vi "LoadCommCfg.vi"(8 "error in (no error)":errorcluster, 10 "section (server name)":string, 11 "Server in":refnum<class "Server.lvclass">) -> (0 "error out":errorcluster, 3 "Server out":refnum<class "Server.lvclass">)   [LabVIEW 2018, in "Server.lvclass"]
uses:
  Server.lvclass
  Server.lvclass/Server.ctl
  <vilib>/Utility/config.llb/Read Key (I32).vi
  <vilib>/Utility/config.llb/Read Key (String).vi
  Comm/Stream/Stream.lvclass
  <vilib>/Utility/config.llb/NI_LVConfig.lvlib
panel:
  out "error commfile2":errorcluster
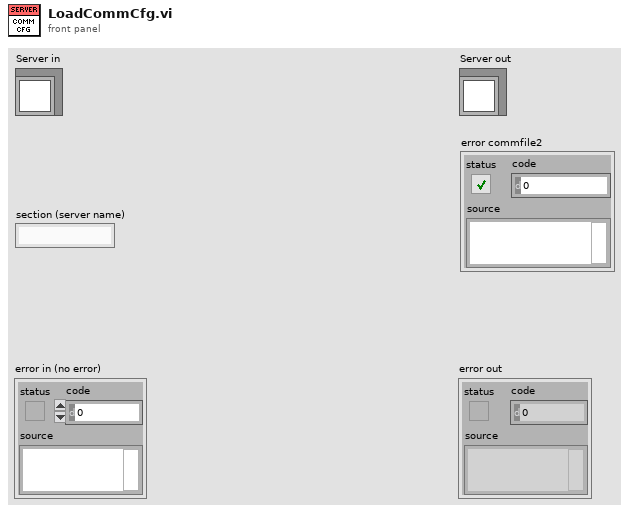
[diagram p1: front panel]
types:
  T1 = typedef "NI_LVConfig.lvlib/Config Data RefNum.ctl" = refnum<k1>
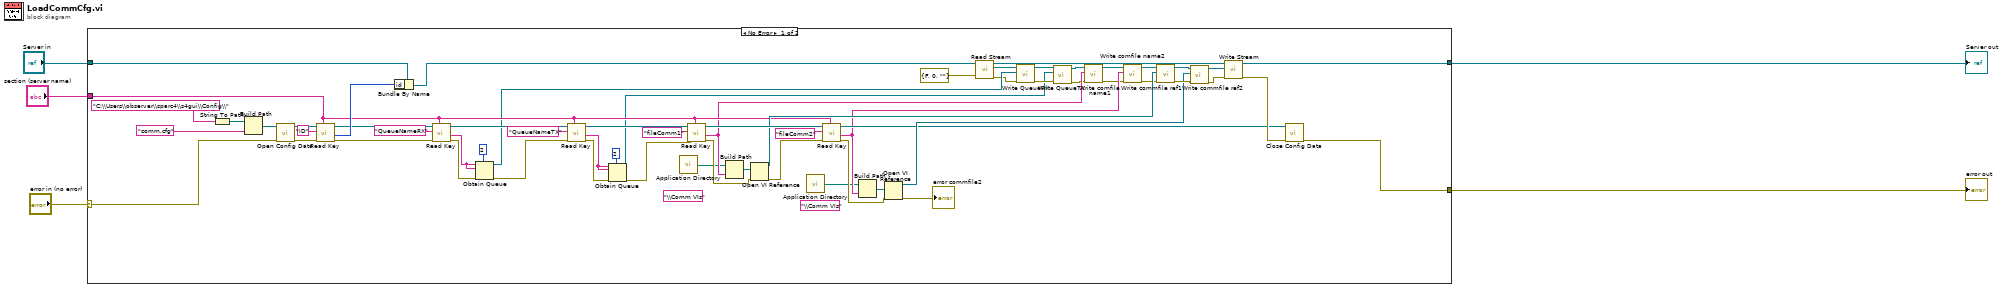
[diagram p0: block diagram]
diagram:
  n1 = case shown="No Error" "error in (no error)" {
    selector: "error in (no error)" -> [w63 w70]
    tunnel: [w60 w70] -> w4
    tunnel: [w48 w69] -> w2
    tunnel: "Server in" -> [w62 w69]
    tunnel: "section (server name)" -> [w31 _]
    frame No Error {
      (unwired) "\\Comm VIs" ("string")
      (unwired) "\\Comm VIs" ("string")
      n2 = String To Path(string="C:\\Users\\observer\\sparc4\\s4gui\\Config\\") -> (path=w6:path)
      n3 = Build Path(base path=w6, name or relative path="comm.cfg") -> (appended path=w68:path)
      n4 = call <vilib>:"Open Config Data.vi"("error in (no error)"=w63, "configuration file path"=w68) -> ("error out"=w65:errorcluster, "refnum"=w67:T1)  [unwired: 7 in, 1 out]
      n5 = call-poly <vilib>:"Read Key.vi"("section"=w31, "error in (no error)"=w65, "key"="ID", "refnum"=w67) -> ("error out"=w51:errorcluster, "value"=w61:i32, "refnum out"=w52:T1)  [unwired: 4 in, 1 out]
      n6 = Bundle By Name(cluster=w62, "id"=w61) -> (w50:refnum<class "Server.lvclass">)
      n7 = call-poly <vilib>:"Read Key.vi"("section"=w31, "error in (no error)"=w51, "key"="QueueNameRX", "refnum"=w52) -> ("error out"=w46:errorcluster, "value"=w58:string, "refnum out"=w57:T1)  [unwired: 4 in, 1 out]
      n8 = Obtain Queue(max queue size (-1, unlimited)=2, name (unnamed)=w58, element data type=w58, error in (no error)=w46) -> (queue out=w18:refnum<queue>, error out=w45:errorcluster)  [unwired: 1 in, 1 out]
      n9 = call-poly <vilib>:"Read Key.vi"("section"=w31, "error in (no error)"=w45, "key"="QueueNameTX", "refnum"=w57) -> ("error out"=w44:errorcluster, "value"=w59:string, "refnum out"=w20:T1)  [unwired: 4 in, 1 out]
      n10 = Obtain Queue(max queue size (-1, unlimited)=2, name (unnamed)=w59, element data type=w59, error in (no error)=w44) -> (queue out=w12:refnum<queue>, error out=w35:errorcluster)  [unwired: 1 in, 1 out]
      n11 = call <vilib>:"Application Directory.vi"() -> ("Application Directory"=w9:path)
      n12 = call-poly <vilib>:"Read Key.vi"("section"=w31, "error in (no error)"=w35, "key"="fileComm1", "refnum"=w20) -> ("error out"=w34:errorcluster, "value"=w26:string, "refnum out"=w43:T1)  [unwired: 4 in, 1 out]
      n13 = Build Path(base path=w9, name or relative path=w26) -> (appended path=w36:path)
      n14 = Open VI Reference(vi path=w36, error in (no error)=w34) -> (vi reference=w32:refnum<vi>, error out=w33:errorcluster)  [unwired: 4 in]
      n15 = call <vilib>:"Application Directory.vi"() -> ("Application Directory"=w8:path)
      n16 = call-poly <vilib>:"Read Key.vi"("section"=w31, "error in (no error)"=w33, "key"="fileComm2", "refnum"=w43) -> ("error out"=w29:errorcluster, "value"=w25:string, "refnum out"=w27:T1)  [unwired: 4 in, 1 out]
      n17 = Build Path(base path=w8, name or relative path=w25) -> (appended path=w30:path)
      n18 = Open VI Reference(vi path=w30, error in (no error)=w29) -> (vi reference=w28:refnum<vi>, error out=→"error commfile2":errorcluster)  [unwired: 4 in]
      n19 = call-dynamic "Read Stream.vi"("error in (no error)"=errorcluster {"status"=FALSE, "code"=0, "source"=""}, "Server in"=w50) -> ("error out"=w17:errorcluster, "Stream.lvclass"=w19:refnum<class "Stream.lvclass">, "Server out"=w49:refnum<class "Server.lvclass">)  [unwired: 7 in]
      n20 = call-dynamic "Write QueueRX.vi"("error in (no error)"=w17, "queue RX"=w18, "Stream in"=w19) -> ("error out"=w15:errorcluster, "Stream out"=w16:refnum<class "Stream.lvclass">)  [unwired: 7 in]
      n21 = call-dynamic "Write QueueTX.vi"("error in (no error)"=w15, "queue TX"=w12, "Stream in"=w16) -> ("error out"=w13:errorcluster, "Stream out"=w14:refnum<class "Stream.lvclass">)  [unwired: 7 in]
      n22 = call-dynamic "Write comfile name1.vi"("error in (no error)"=w13, "comfile name1"=w26, "Stream in"=w14) -> ("error out"=w22:errorcluster, "Stream out"=w24:refnum<class "Stream.lvclass">)  [unwired: 7 in]
      n23 = call-dynamic "Write comfile name2.vi"("error in (no error)"=w22, "comfile name2"=w25, "Stream in"=w24) -> ("error out"=w21:errorcluster, "Stream out"=w23:refnum<class "Stream.lvclass">)  [unwired: 7 in]
      n24 = call-dynamic "Write commfile ref1.vi"("error in (no error)"=w21, "commfile ref1"=w32, "Stream in"=w23) -> ("error out"=w38:errorcluster, "Stream out"=w40:refnum<class "Stream.lvclass">)  [unwired: 7 in]
      n25 = call-dynamic "Write commfile ref2.vi"("error in (no error)"=w38, "commfile ref2"=w28, "Stream in"=w40) -> ("error out"=w37:errorcluster, "Stream out"=w39:refnum<class "Stream.lvclass">)  [unwired: 7 in]
      n26 = call-dynamic "Write Stream.vi"("error in (no error)"=w37, "Stream.lvclass"=w39, "Server in"=w49) -> ("error out"=w47:errorcluster, "Server out"=w48:refnum<class "Server.lvclass">)  [unwired: 7 in]
      n27 = call <vilib>:"Close Config Data.vi"("error in (no error)"=w47, "refnum"=w27) -> ("error out"=w60:errorcluster)  [unwired: 8 in, 1 out]
    }
    frame Error {
    }
  }
  "error out" <- w4
  "Server out" <- w2
